vi "write line in table.vi"(8 "error in":errorcluster, 9 "line":T1, 10 "line number":i32, 11 "operations table":T2) -> (0 "error out":errorcluster)   [LabVIEW 2013, in "TEC editor node.lvclass"]
uses:
  TEC editor node.lvclass
  table reference.ctl
  table line.ctl
  <vilib>/NI/Tag Bus Module Framework/channel/TBM channel.lvclass
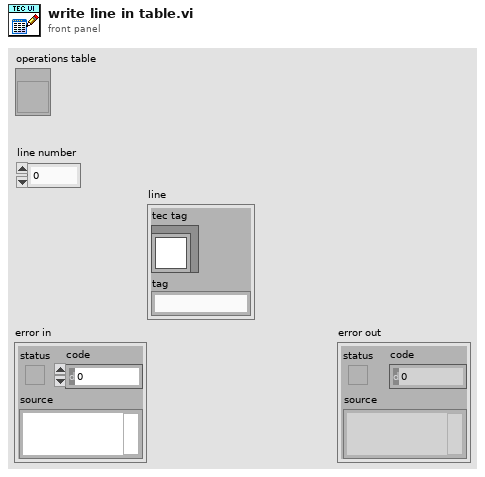
[diagram p1: front panel]
types:
  T1 = typedef "TEC editor node.lvclass/table line.ctl" = cluster{"tec tag":refnum<class "TBM channel.lvclass">, "tag":string}
  T2 = typedef "TEC editor node.lvclass/table reference.ctl" = refnum<vi>
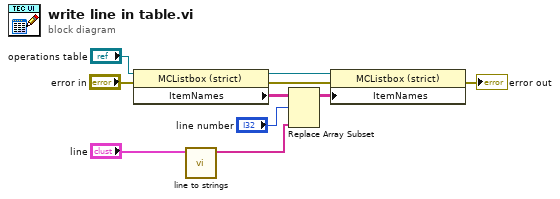
[diagram p0: block diagram]
diagram:
  n1 = property class="MCListbox (strict)"(reference="operations table", error in="error in") -> (reference out=w5:T2, error out=w8:errorcluster, "ItemNames"=w4:string[][])
  n2 = call "line to strings.vi"("line"="line") -> ("strings"=w2:string[])  [unwired: 10 in]
  n3 = Replace Array Subset(array=w4, new element=w2, index (row)="line number") -> (w3:string[][])  [unwired: 1 in]
  n4 = property class="MCListbox (strict)"(reference=w5, error in=w8, "ItemNames"=w3) -> (error out=→"error out":errorcluster)  [unwired: 1 out]
